vi "oa_SCL Draw Plot.vi"(4 "y scale factors":cluster{"a":dbl, "b":dbl, "log?":bool} {"b" format="%0.2f"; "a" format="%0.2f"}, 5 "XY plot cosmetics":T2={"plot color"=16776960, "XY plot type"=enum."connected points", "baseline"=0.0} {"baseline" format="%0.2f"}, 6 "x scale factors":cluster{"a":dbl, "b":dbl, "log?":bool} {"b" format="%0.2f"; "a" format="%0.2f"}, 10 "data":cluster{"x":dbl, "y":dbl}[](array[cluster]) {"y" format="%0.2f"; "x" format="%0.2f"}, 11 "picture":picture) -> (3 "new picture":picture)   [LabVIEW 2017]
uses:
  <vilib>/picture/cartesn2.llb/XY Plot Type.ctl
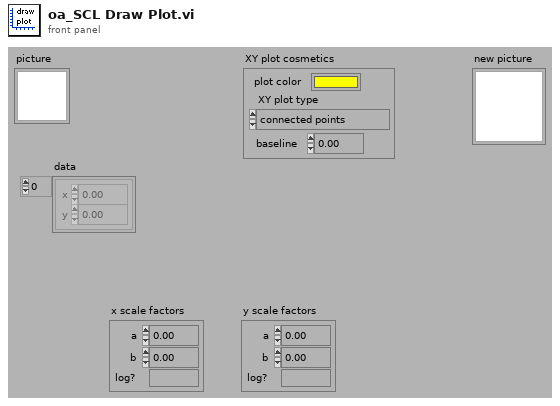
[diagram p1: front panel]
types:
  T1 = typedef "XY Plot Type.ctl" = enum16{"points", "squares", "circles", "connected points", "connected squares", "connected circles", "comb plot", "sized scatter plot", "sized-colored scatter plot", "min-max lines"}
  T2 = cluster{"plot color":u32, "XY plot type":T1, "baseline":dbl}
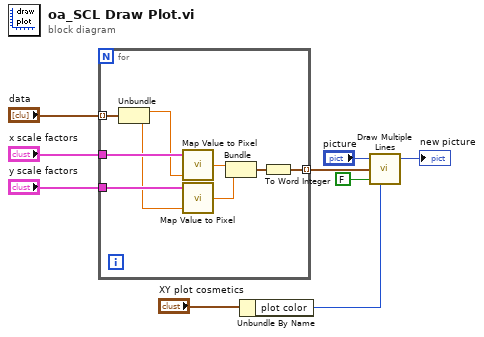
[diagram p0: block diagram]
diagram:
  n1 = for {
    tunnel: "data" -> [w18] mode=indexing
    tunnel: "x scale factors" -> [w17]
    tunnel: "y scale factors" -> [w15]
    tunnel: [w10] -> w1 mode=indexing
    n2 = Unbundle(w18) -> ("x"=w16:dbl, "y"=w14:dbl)
    n3 = call <vilib>:"Map Value to Pixel.vi"("x"=w16, "scale factors"=w17) -> ("pixel"=w13:dbl)  [unwired: 1 in]
    n4 = call <vilib>:"Map Value to Pixel.vi"("x"=w14, "scale factors"=w15) -> ("pixel"=w12:dbl)  [unwired: 1 in]
    n5 = Bundle("pixel"=w13, "pixel"=w12) -> (w11:cluster{"pixel":dbl, "pixel":dbl})  [unwired: 1 in]
    n6 = To Word Integer(number=w11) -> (16bit integer=w10:cluster{"pixel":i16, "pixel":i16})
  }
  n7 = Unbundle By Name("XY plot cosmetics") -> ("plot color"=w3:u32)
  n8 = call <vilib>:"Draw Multiple Lines.vi"("picture"="picture", "line endpoints"=w1, "fill?(F)"=FALSE, "color(black)"=w3) -> ("new picture"=→"new picture":picture)  [unwired: 5 in]
